vi "Calculate_T_to_H2O_LBSperGAL.vi"(10 "Termperature":dbl format="%_6g") -> (2 "lbs/Gal":dbl)   [LabVIEW 2013]
uses:
  <vilib>/gmath/NI_Gmath.lvlib
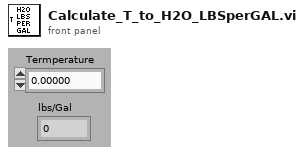
[diagram p1: front panel]
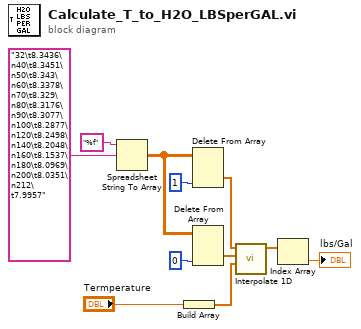
[diagram p0: block diagram]
diagram:
  n1 = Spreadsheet String To Array(format string="%f", spreadsheet string="32\t8.3436\n40\t8.3451\n50\t8.343\n60\t8.3378\n70\t8.329\n80\t8.3176\n90\t8.3077\n100\t8.2877\n120\t8.2498\n140\t8.2048\n160\t8.1537\n180\t8.0969\n200\t8.0351\n212\t7.9957") -> (array=w7:dbl[][])  [unwired: 2 in]
  n2 = Build Array("Termperature") -> (w3:dbl[])
  n3 = Delete From Array(array=w7, index (col)=1 ("disabled index (col)")) -> (deleted portion=w8:dbl[])  [unwired: 2 in, 1 out]
  n4 = Delete From Array(array=w7, index (col)=0 ("disabled index (col)")) -> (deleted portion=w5:dbl[])  [unwired: 2 in, 1 out]
  n5 = call <vilib>:"Interpolate 1D.vi"("xi"=w3, "X"=w5, "Y"=w8) -> ("yi"=w2:dbl[])  [unwired: 6 in, 2 out]
  n6 = Index Array(array=w2) -> (element=→"lbs/Gal":dbl)  [unwired: 1 in]
